vi "RTMain.vi"() -> ()   [LabVIEW 2014]
uses:
  <vilib>/Modbus/slave/Create Slave Instance (TCP).vi
  <vilib>/Modbus/slave/Modbus Slave.lvclass
panel:
  out "Array 3":u16[](array[numeric])
  in  "UTC format":bool
  out "Array":u16[](array[numeric])
  out "TCP Connection List":T1(array[cluster])
  in  "time format string (%c)":string="%Y %m %d %H %M %S"
  in  "Stop":bool
  out "Number of Masters":u32
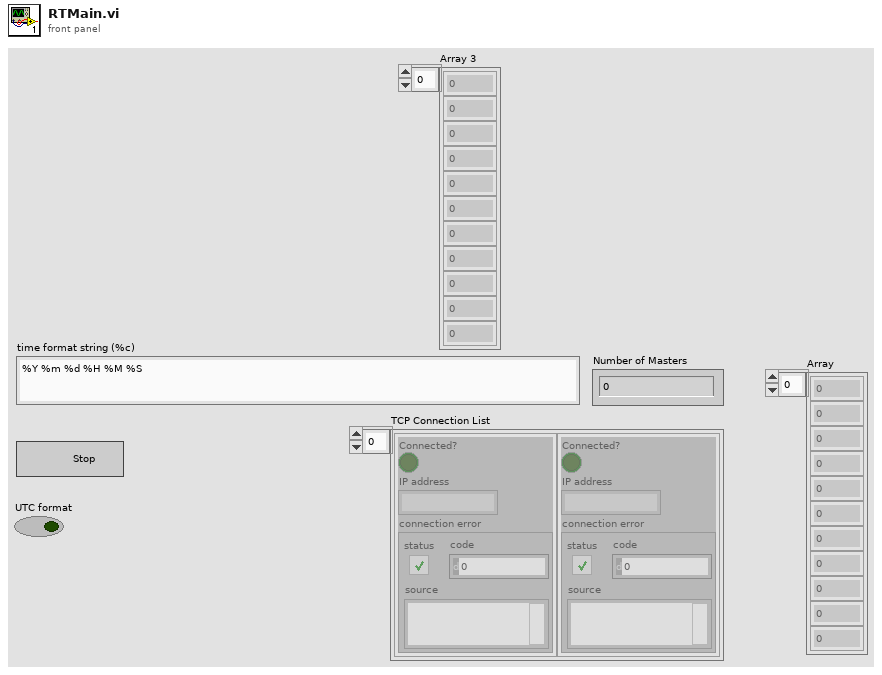
[diagram p1: front panel]
types:
  T1 = cluster{"Connected?":bool, "IP address":string, "connection error":errorcluster}[]
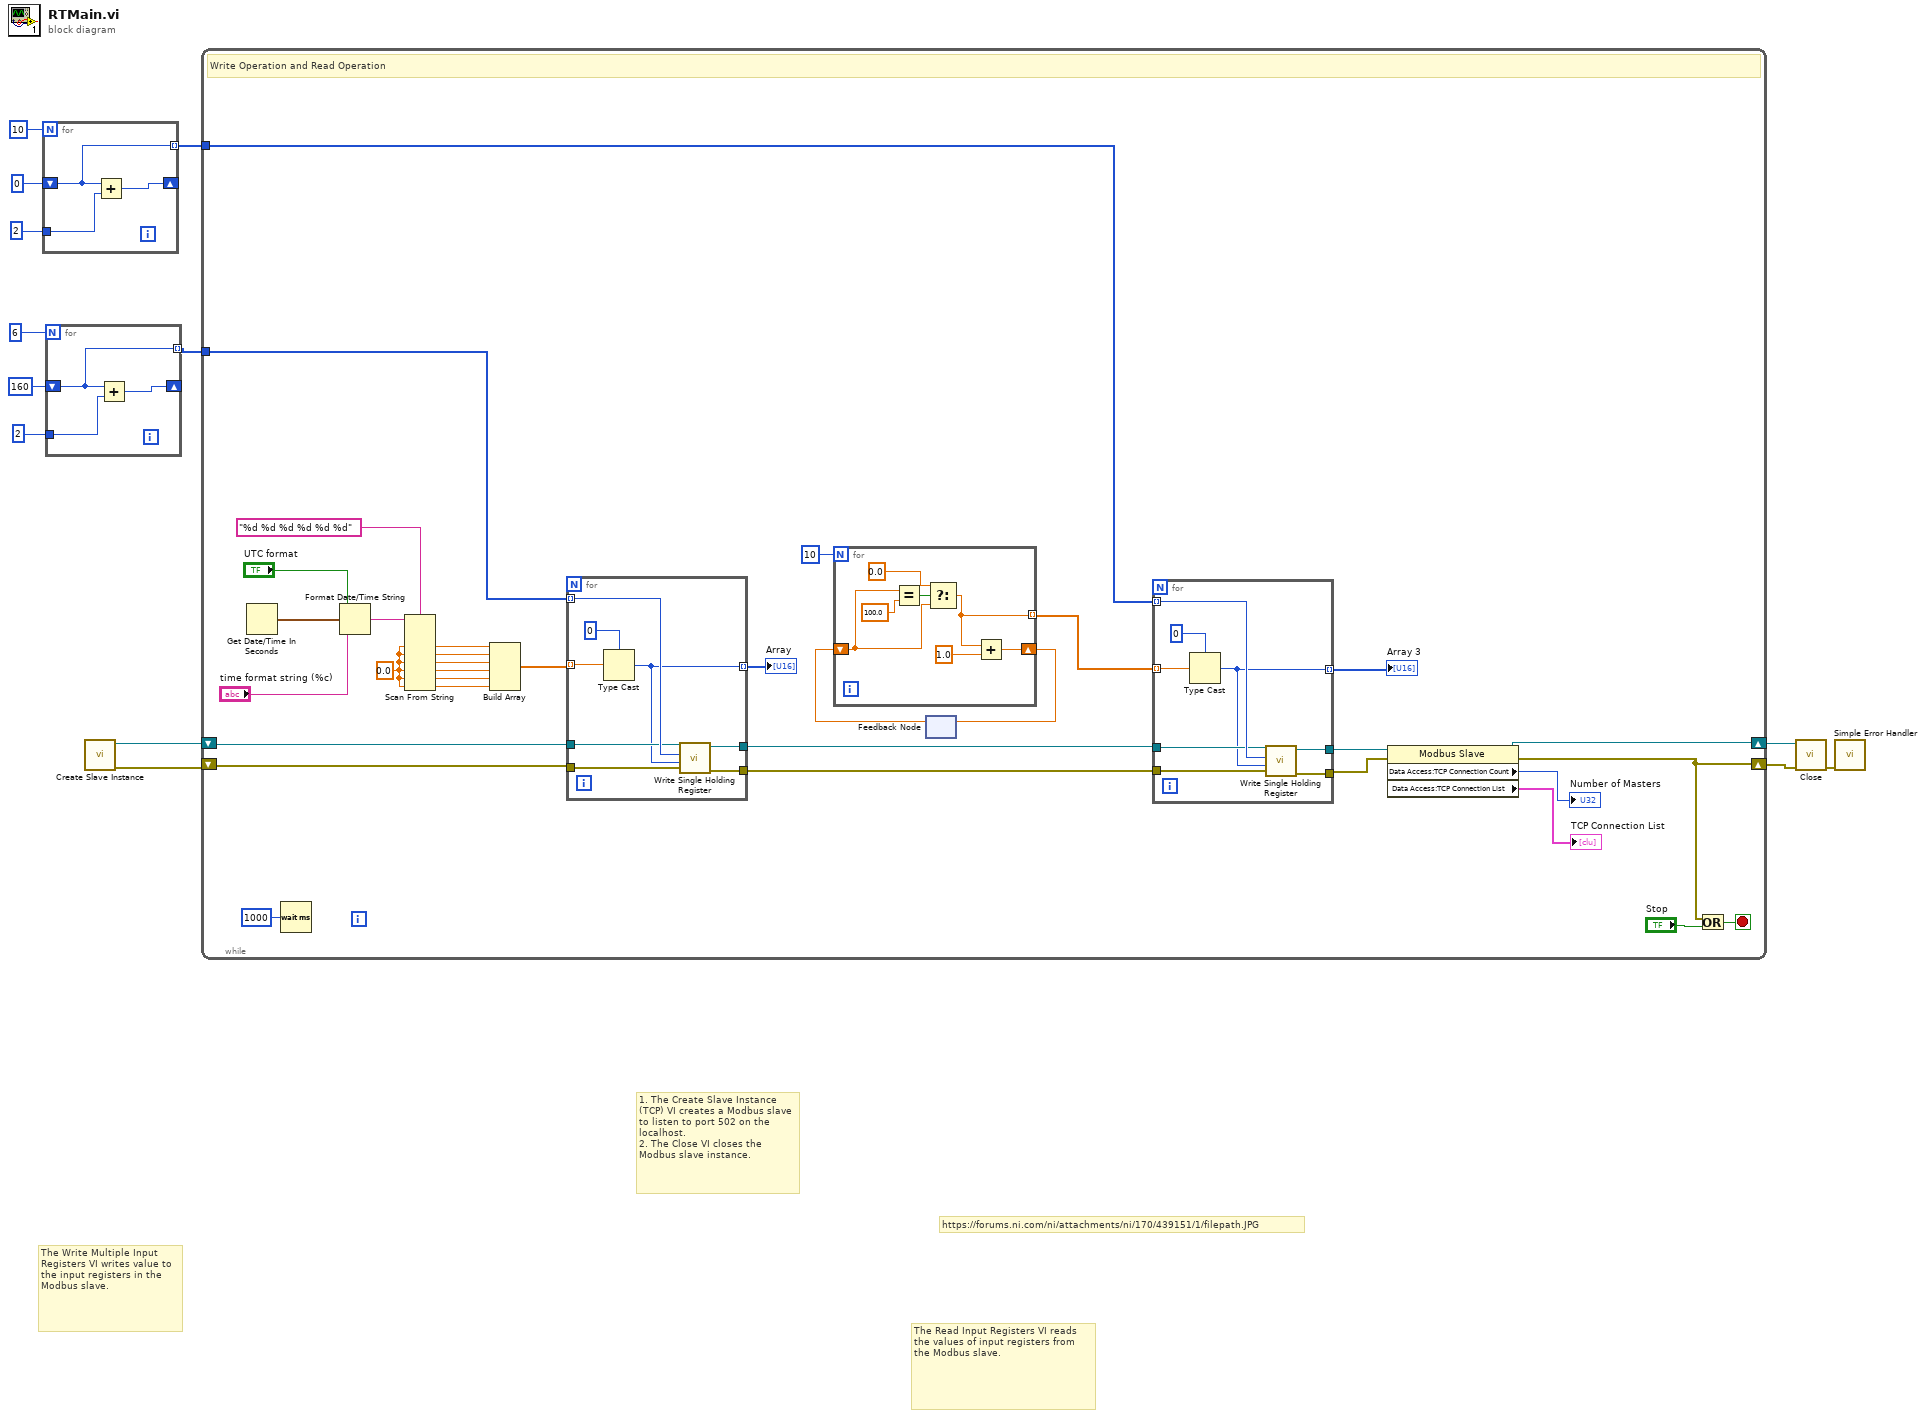
[diagram p0: block diagram]
diagram:
  # "https://forums.ni.com/ni/attachments/ni/170/439151/1/filepath.JPG"
  # "The Read Input Registers VI reads the values of input registers from the Modbus slave."
  # "The Write Multiple Input Registers VI writes value to the input registers in the Modbus slave."
  # "1. The Create Slave Instance (TCP) VI creates a Modbus slave to listen to port 502 on the localhost.\n2. The Close VI closes the Modbus slave instance."
  n1 = for {
    N: 10 -> [_]
    tunnel: u16 2 ("y") -> [w16]
    shift-right: [w15] -> _
    shift-left: u16 0 ("holding register value") -> [w14]
    tunnel: [w14] -> w1 mode=indexing
    n2 = Add(x=w14, y=w16) -> (x+y=w15:u16)
  }
  n3 = for {
    N: 6 -> [_]
    tunnel: u16 2 ("y") -> [w19]
    shift-right: [w18] -> _
    shift-left: u16 160 ("holding register value") -> [w17]
    tunnel: [w17] -> w5 mode=indexing
    n4 = Add(x=w17, y=w19) -> (x+y=w18:u16)
  }
  n5 = call-poly <vilib>:"Create Slave Instance.vi"() -> ("error out"=w9:errorcluster, "TCP slave instance"=w13:refnum<class "Modbus Slave.lvclass">)  [unwired: 10 in]
  n6 = while {
    shift-right: [w50] -> w11
    shift-left: w13 -> [w37]
    shift-right: [w49] -> w12
    shift-left: w9 -> [w36]
    tunnel: w5 -> [w25]
    tunnel: w1 -> [w24]
    stop <- w51 stop-if-true
    w34 = sgl 0.0 ("default value 1")
    # "Write Operation and Read Operation"
    n7 = Get Date/Time In Seconds() -> (seconds since 1Jan1904=w47:timestamp)
    n8 = Wait (ms)(milliseconds to wait=u32 1000) -> ()  [unwired: 1 out]
    n9 = Format Date/Time String(time format string (%c)="time format string (%c)", seconds (now)=w47, UTC format="UTC format") -> (date/time string=w45:string)
    n10 = Scan From String(format string="%d %d %d %d %d %d", input string=w45, default 1=w34, default 2=w34, default 3=w34, default 4=w34, default 5=w34, default 6=w34) -> (output 1=w31:sgl, output 2=w43:sgl, output 3=w42:sgl, output 4=w41:sgl, output 5=w40:sgl, output 6=w39:sgl)  [unwired: 2 in, 3 out]
    n11 = Build Array(w31, w43, w42, w41, w40, w39) -> (w35:sgl[])
    n12 = for {
      tunnel: w37 -> [w74]
      tunnel: w36 -> [w75]
      tunnel: w25 -> [w76] mode=indexing
      tunnel: [w73] -> w27
      tunnel: [w72] -> w28
      tunnel: w35 -> [w70] mode=indexing
      tunnel: [w69] -> w33 mode=indexing
      n13 = Type Cast(type=u16 0, x=w70) -> (*(type *) &x=w69:u16)
      n14 = call-dynamic "Write Single Holding Register.vi"("error in (no error)"=w75, "holding register value"=w69, "address"=w76, "Modbus slave in"=w74) -> ("error out"=w72:errorcluster, "Modbus slave out"=w73:refnum<class "Modbus Slave.lvclass">)  [unwired: 6 in]
    }
    "Array" <- w33
    n15 = feedback #1() -> (w23:sgl)  [unwired: 1 in]
    n16 = for {
      N: 10 -> [_]
      tunnel: [w55] -> w20 mode=indexing
      shift-right: [w59] -> w21
      shift-left: w23 -> [w56]
      n17 = Equal?(x=w56, y=sgl 100.0) -> (x = y?=w57:bool)
      n18 = Select(t=sgl 0.0 ("y"), s=w57, f=w56) -> (s? t:f=w55:sgl)
      n19 = Add(x=w55, y=sgl 1.0) -> (x+y=w59:sgl)
    }
    n20 = feedback-in #1(w21) -> ()
    n21 = for {
      tunnel: w27 -> [w66]
      tunnel: w28 -> [w67]
      tunnel: w24 -> [w68] mode=indexing
      tunnel: [w65] -> w26
      tunnel: [w64] -> w29
      tunnel: [w62] -> w30 mode=indexing
      tunnel: w20 -> [w61] mode=indexing
      n22 = Type Cast(type=u16 0, x=w61) -> (*(type *) &x=w62:u16)
      n23 = call-dynamic "Write Single Holding Register.vi"("error in (no error)"=w67, "holding register value"=w62, "address"=w68, "Modbus slave in"=w66) -> ("error out"=w64:errorcluster, "Modbus slave out"=w65:refnum<class "Modbus Slave.lvclass">)  [unwired: 6 in]
    }
    "Array 3" <- w30
    n24 = property class="Modbus Slave"(reference=w26, error in=w29) -> (reference out=w50:refnum<class "Modbus Slave.lvclass">, error out=w49:errorcluster, "Data Access:TCP Connection Count"=→"Number of Masters":u32, "Data Access:TCP Connection List"=→"TCP Connection List":T1)
    n25 = Or(x=w49, y="Stop") -> (x .or. y?=w51:bool)
  }
  n26 = call-dynamic "Close.vi"("error in (no error)"=w12, "Modbus slave in"=w11) -> ("error out"=w10:errorcluster)  [unwired: 9 in]
  n27 = call <vilib>:"Simple Error Handler.vi"("error in (no error)"=w10) -> ()  [unwired: 4 in, 5 out]
